vi "PruebaSequence.vi"() -> ()   [LabVIEW 2014, in "MSX-E3701.lvlib"]
uses:
  MSX-E3701.lvlib
  MSX-E3701Class/MSX-E3701.lvclass
panel:
  out "TDX":sgl[][](array[numeric]) format="%#.5f"
  out "Muestras por seg":dbl
  out "Segundos":dbl
  out "Muestras":i32
  out "error out":errorcluster
  in  "stop":bool
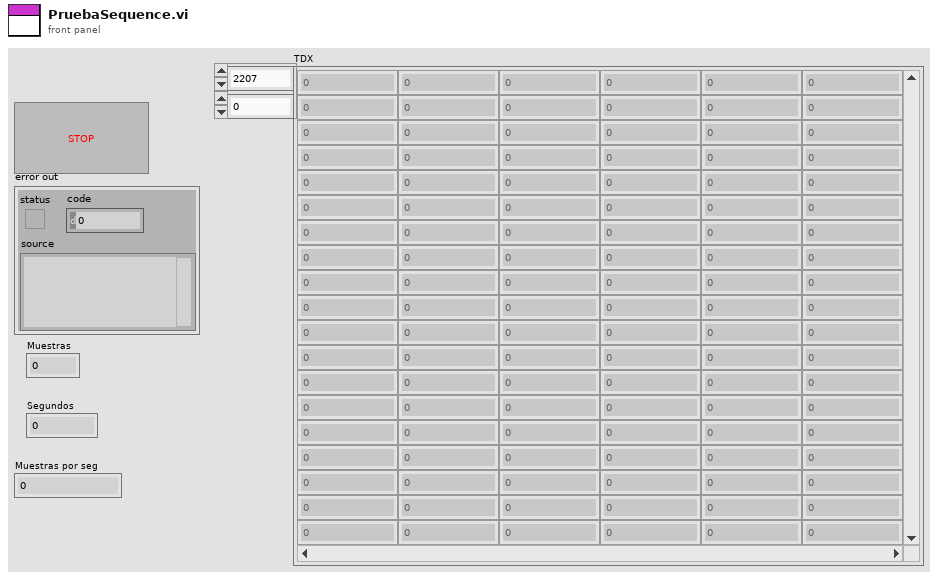
[diagram p1: front panel]
types:
  T1 = typedef "DriverMasterSync.lvlibp/WINFAS 2 Data Queue.lvlib/Control Data Cluster.ctl" = cluster{"Encoder":sgl, "DI":bool[], "DO":bool[]}
  T2 = typedef "DriverMasterSync.lvlibp/WINFAS 2 Data Queue.lvlib/Acquisition Data Cluster.ctl" = T3[]
  T3 = typedef "DriverMasterSync.lvlibp/WINFAS 2 Data Queue.lvlib/Acquisition Data 1 Sample Cluster.ctl" = cluster{"TDX":sgl[], "Encoder":sgl}
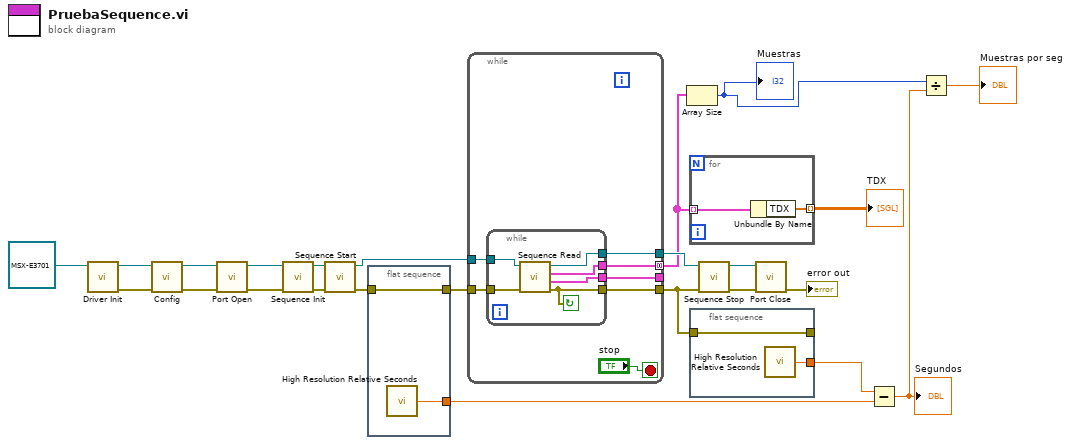
[diagram p0: block diagram]
diagram:
  n1 = call-dynamic "Driver Init.vi"("MSX-E3701 in"=refnum<class "MSX-E3701.lvclass"> refnum) -> ("error out"=w3:errorcluster, "MSX-E3701 out"=w2:refnum<class "MSX-E3701.lvclass">)  [unwired: 9 in]
  n2 = call-dynamic "Config.vi"("error in (no error)"=w3, "MSX-E3701 in"=w2) -> ("error out"=w24:errorcluster, "MSX-E3701 out"=w15:refnum<class "MSX-E3701.lvclass">)  [unwired: 7 in, 1 out]
  n3 = call-dynamic "Port Open.vi"("error in (no error)"=w24, "MSX-E3701 in"=w15) -> ("error out"=w23:errorcluster, "MSX-E3701 out"=w16:refnum<class "MSX-E3701.lvclass">)  [unwired: 8 in]
  n4 = call-dynamic "Sequence Init.vi"("error in (no error)"=w23, "MSX-E3701 in"=w16) -> ("error out"=w22:errorcluster, "MSX-E3701 out"=w17:refnum<class "MSX-E3701.lvclass">)  [unwired: 8 in]
  n5 = call-dynamic "Sequence Start.vi"("error in (no error)"=w22, "MSX-E3701 in"=w17) -> ("error out"=w13:errorcluster, "MSX-E3701 out"=w18:refnum<class "MSX-E3701.lvclass">)  [unwired: 8 in]
  n6 = flat-sequence {
    tunnel: [w26] -> w12
    tunnel: w13 -> [w26]
    tunnel: [w25] -> w9
    frame #0 {
      n7 = call <vilib>:"High Resolution Relative Seconds.vi"() -> ("relative seconds"=w25:dbl)
    }
  }
  n8 = while {
    tunnel: w12 -> [w33]
    tunnel: [w32] -> w11
    tunnel: w18 -> [w30]
    tunnel: [w31] -> w19
    tunnel: [w28] -> w5 mode=concatenating
    tunnel: [w27] -> _
    stop <- "stop" stop-if-true
    n9 = while {
      tunnel: w33 -> [w39]
      tunnel: [w36] -> w32
      tunnel: w30 -> [w37]
      tunnel: [w38] -> w31
      tunnel: [w35] -> w28
      tunnel: [w34] -> w27
      stop <- w36 continue-if-true
      n10 = call-dynamic "Sequence Read.vi"("error in (no error)"=w39, "MSX-E3701 in"=w37) -> ("error out"=w36:errorcluster, "Control Data"=w34:T1, "Acquisition Data"=w35:T2, "MSX-E3701 out"=w38:refnum<class "MSX-E3701.lvclass">)  [unwired: 6 in]
    }
  }
  n11 = Array Size(array=w5) -> (size(s)=w4:i32)
  "Muestras" <- w4
  n12 = for {
    tunnel: w5 -> [w41] mode=indexing
    tunnel: [w40] -> w6 mode=indexing
    n13 = Unbundle By Name(w41) -> ("TDX"=w40:sgl[])
  }
  "TDX" <- w6
  n14 = flat-sequence {
    tunnel: [w43] -> _
    tunnel: w11 -> [w43]
    tunnel: [w42] -> w10
    frame #0 {
      n15 = call <vilib>:"High Resolution Relative Seconds.vi"() -> ("relative seconds"=w42:dbl)
    }
  }
  n16 = call-dynamic "Sequence Stop.vi"("error in (no error)"=w11, "MSX-E3701 in"=w19) -> ("error out"=w21:errorcluster, "MSX-E3701 out"=w20:refnum<class "MSX-E3701.lvclass">)  [unwired: 8 in]
  n17 = call-dynamic "Port Close.vi"("error in (no error)"=w21, "MSX-E3701 in"=w20) -> ("error out"=→"error out":errorcluster)  [unwired: 8 in, 1 out]
  n18 = Subtract(x=w10, y=w9) -> (x-y=w8:dbl)
  "Segundos" <- w8
  n19 = Divide(x=w4, y=w8) -> (x/y=→"Muestras por seg":dbl)
